vi "MFCConfigurationGlobal.vi"(5 "Index":u16, 7 "Action":T5=enum."Get", 8 "Error In":errorcluster, 11 "Set Value":T1) -> (0 "Error Out":errorcluster, 3 "Value Out":T1)   [LabVIEW 2012]
uses:
  MFCConfigurationGlobalAction.ctl
  MFCConfiguration.ctl
  libs/Sierra-M100/Public/Controls/ValveState.ctl
  libs/Sierra-M100/Public/Controls/Gas.ctl
  libs/Sierra-M100/Public/Controls/Units.ctl
  libs/Sierra-M100/Sierra-M100.lvlib
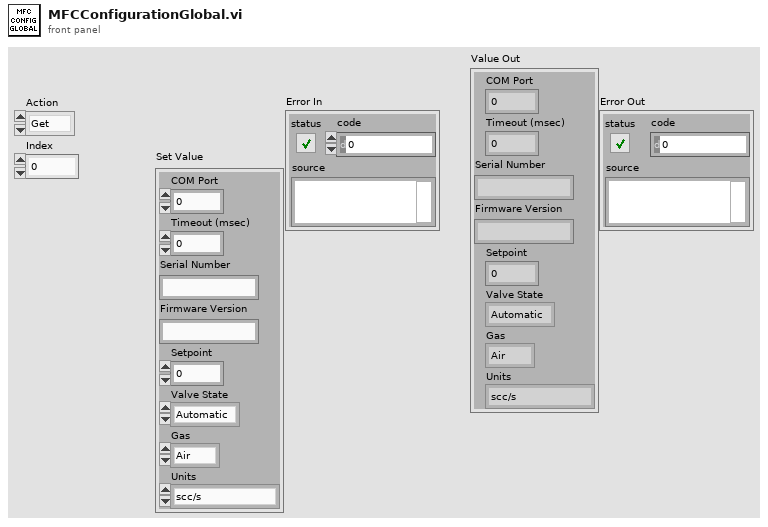
[diagram p1: front panel]
types:
  T1 = typedef "MFCConfiguration.ctl" = cluster{"COM Port":u32, "Timeout (msec)":u32, "Setpoint":dbl, "Valve State":T2, "Gas":T3, "Units":T4, "Serial Number":string, "Firmware Version":string}
  T2 = typedef "Sierra-M100.lvlib/ValveState.ctl" = enum16{"Automatic", "Closed", "Purge"}
  T3 = typedef "Sierra-M100.lvlib/Gas.ctl" = enum16{"Air", "Argon", "CO2", "CO", "Helium", "Hydrogen", "Methane", "Nitrogen", "Nitrous Oxide", "Oxygen"}
  T4 = typedef "Sierra-M100.lvlib/Units.ctl" = enum16{"scc/s", "scc/m", "scc/H", "Ncc/s", "Ncc/m", "Ncc/H", "SCF/s", "SCF/m", "SCF/H", "NM3/s", "NM3/m", "NM3/H", "SM3/s", "SM3/m", "SM3/H", "sl/s", "sl/m", "sl/H", "NL/s", "NL/m", "Nl/H", "g/s", "g/m", "g/H", "kg/s", "kg/m", "kg/H", "lb/s", "lb/m", "lb/H"}
  T5 = typedef "MFCConfigurationGlobalAction.ctl" = enum16{"Init", "Get", "Set", "Add", "Remove", "Reset"}
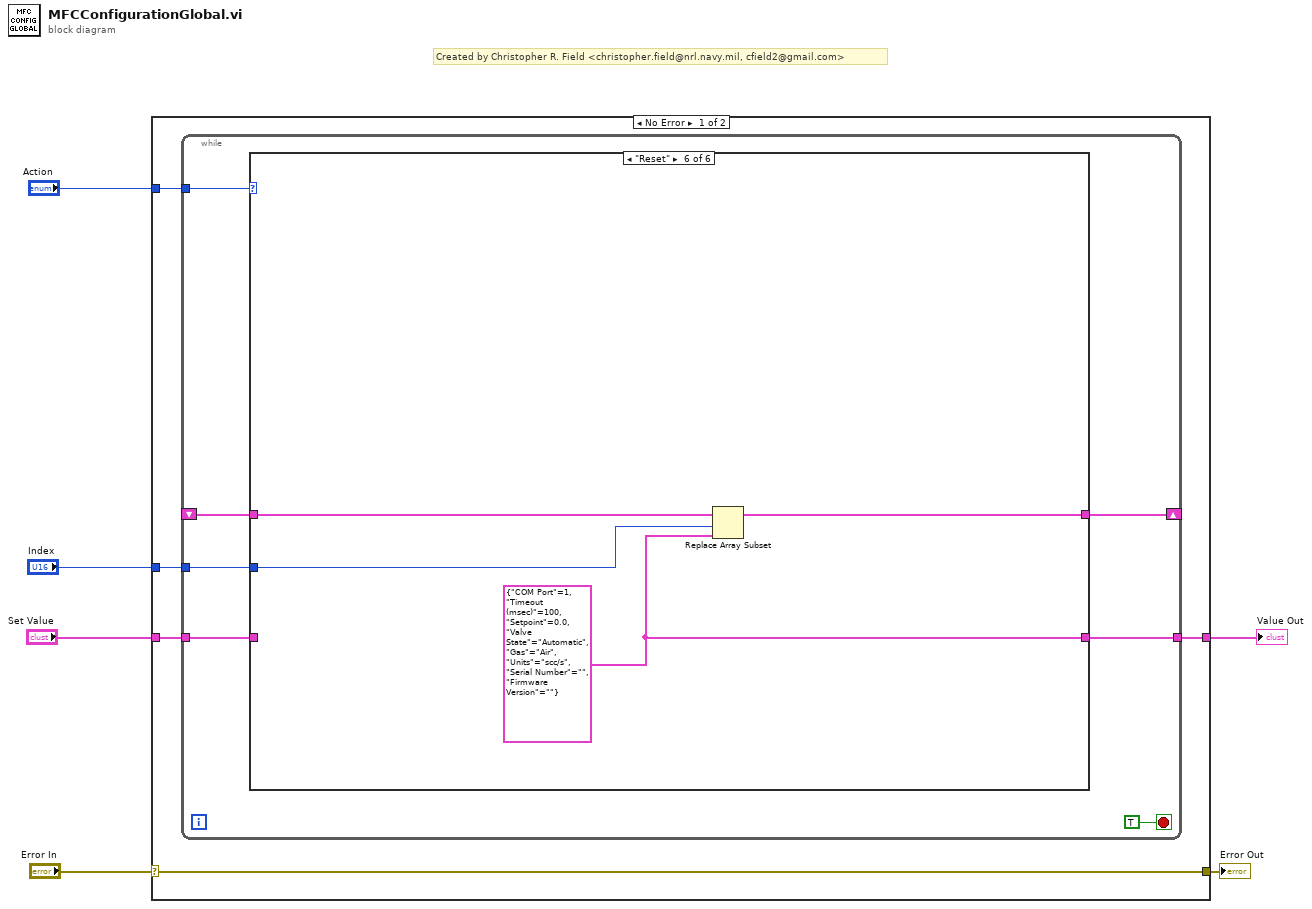
[diagram p0: block diagram]
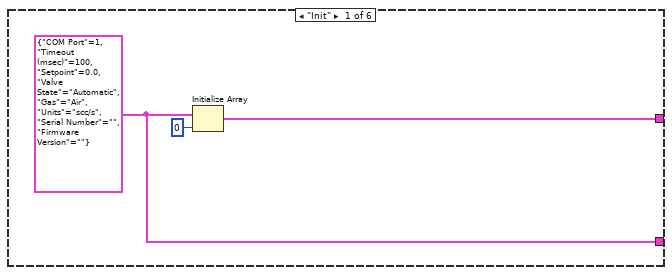
[diagram p2: hidden frame]
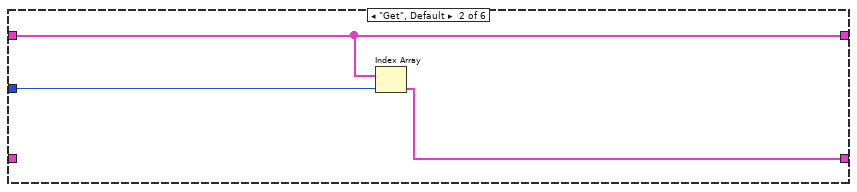
[diagram p3: hidden frame]
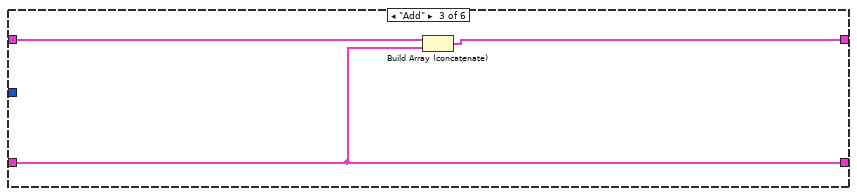
[diagram p4: hidden frame]
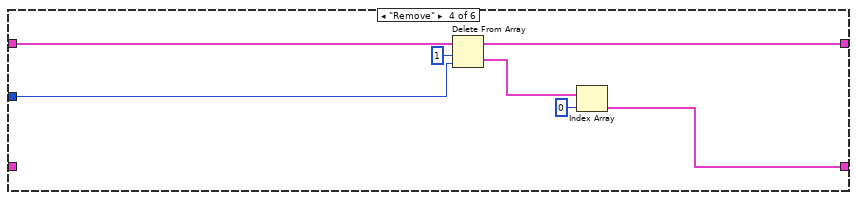
[diagram p5: hidden frame]
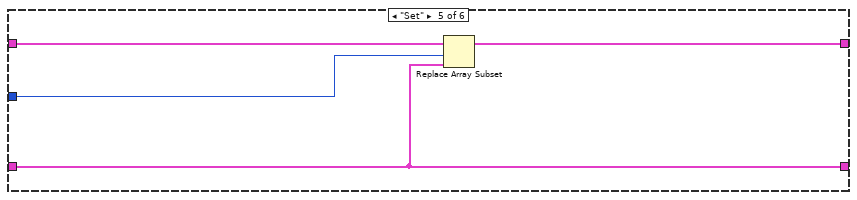
[diagram p6: hidden frame]
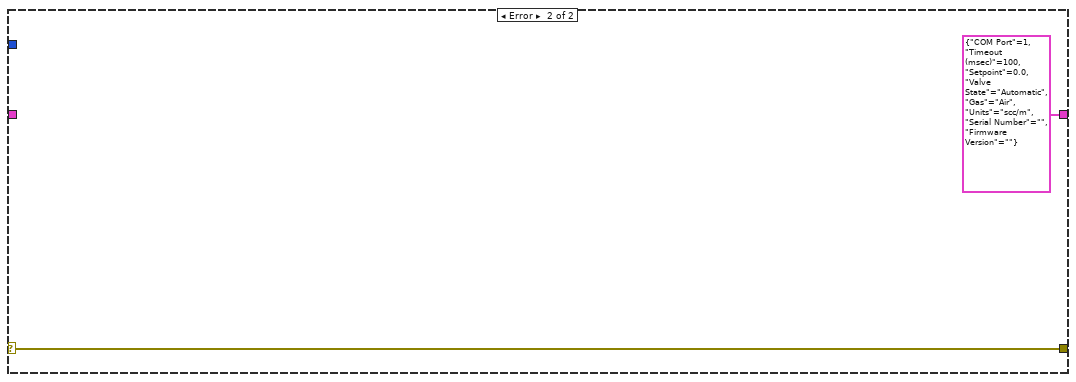
[diagram p7: hidden frame]
diagram:
  # "Created by Christopher R. Field <christopher.field@nrl.navy.mil, cfield2@gmail.com>"
  n1 = case shown="No Error" "Error In" {
    selector: "Error In" -> [w7 w44]
    tunnel: "Action" -> [w11 _]
    tunnel: "Set Value" -> [w10 _]
    tunnel: [w9 T1 {"COM Port"=1, "Timeout (msec)"=100, "Setpoint"=0.0, "Valve State"=enum."Automatic", "Gas"=enum."Air", "Units"=enum."scc/m", "Serial Number"="", "Firmware Version"=""} ("Set Value")] -> w4
    tunnel: "Index" -> [w8 _]
    tunnel: [w7 w44] -> w1
    frame No Error {
      n2 = while {
        tunnel: w11 -> [w17]
        tunnel: w10 -> [w16]
        shift-right: [w14] -> _
        shift-left: _ -> [w15]
        tunnel: [w13] -> w9
        tunnel: w8 -> [w12]
        stop <- TRUE stop-if-true
        n3 = case shown="\"Reset\"" w17 {
          tunnel: w16 -> [_ _ w26 _ w35 _]
          tunnel: w15 -> [_ w24 w27 w34 w38 w42]
          tunnel: [w20 w24 w25 w33 w37 w41] -> w14
          tunnel: [w19 w22 w26 w28 w35 w39] -> w13
          tunnel: w12 -> [_ w23 _ w30 w36 w40]
          frame "Init" {
            w19 = T1 {"COM Port"=1, "Timeout (msec)"=100, "Setpoint"=0.0, "Valve State"=enum."Automatic", "Gas"=enum."Air", "Units"=enum."scc/s", "Serial Number"="", "Firmware Version"=""} ("Set Value")
            n4 = Initialize Array(w19, 0 ("dimension size")) -> (w20:T1[])
          }
          frame "Get", Default {
            n5 = Index Array(array=w24, index=w23) -> (element=w22:T1)
          }
          frame "Add" {
            n6 = Build Array (concatenate)(w27, w26) -> (w25:T1[])
          }
          frame "Remove" {
            n7 = Delete From Array(array=w34, length=1, index=w30) -> (deleted portion=w32:T1[], array with subset deleted=w33:T1[])
            n8 = Index Array(array=w32, index=0) -> (element=w28:T1)
          }
          frame "Set" {
            n9 = Replace Array Subset(array=w38, new element=w35, index=w36) -> (w37:T1[])
          }
          frame "Reset" {
            w39 = T1 {"COM Port"=1, "Timeout (msec)"=100, "Setpoint"=0.0, "Valve State"=enum."Automatic", "Gas"=enum."Air", "Units"=enum."scc/s", "Serial Number"="", "Firmware Version"=""} ("Set Value")
            n10 = Replace Array Subset(array=w42, new element=w39, index=w40) -> (w41:T1[])
          }
        }
      }
    }
    frame Error {
    }
  }
  "Value Out" <- w4
  "Error Out" <- w1
